vi "AVI Video Re-Initialise.vi"() -> (0 "error out":errorcluster)   [LabVIEW 2017]
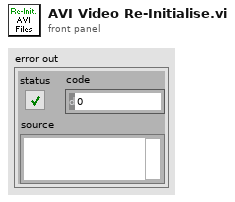
[diagram p1: front panel]
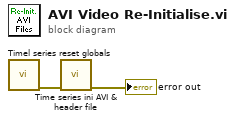
[diagram p0: block diagram]
diagram:
  n1 = call "Timel series reset globals.vi"() -> ("error out"=w2:errorcluster)  [unwired: 11 in]
  n2 = call "Time series ini AVI & header file.vi"("error in (no error)"=w2) -> ("error out"=→"error out":errorcluster)  [unwired: 10 in]
